vi "Pre-Disconnect.vi"(8 "error in":errorcluster, 11 "4300 in":refnum<class "4300.lvclass">) -> (0 "error out":errorcluster, 3 "4300 out":refnum<class "4300.lvclass">)   [LabVIEW 2019, in "4300.lvlib" / "4300.lvclass"]
uses:
  4300.lvclass
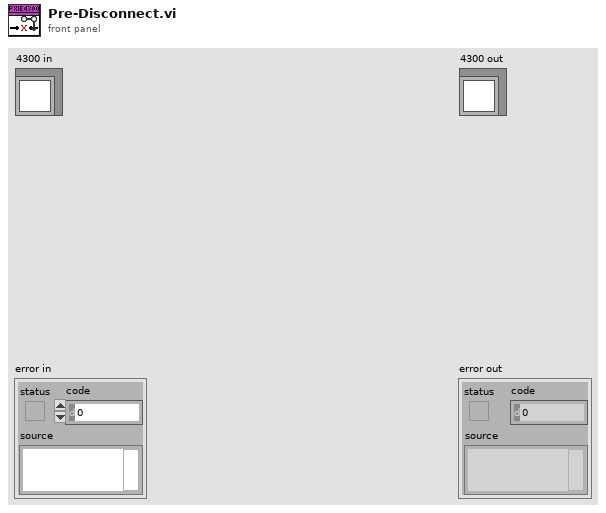
[diagram p1: front panel]
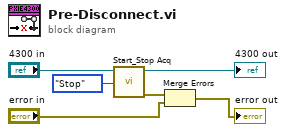
[diagram p0: block diagram]
diagram:
  n1 = call-dynamic "Start_Stop Acq.vi"("Start/Stop"=enum16{"Start", "Stop"}."Stop", "4300 in"="4300 in") -> ("error out"=w4:errorcluster, "4300 out"=→"4300 out":refnum<class "4300.lvclass">)  [unwired: 8 in]
  n2 = Merge Errors(w4, "error in") -> (→"error out":errorcluster)
